vi "Energize.vi"(8 "error in (no error)":errorcluster, 11 "CIFTemplatePlugin in":refnum<class "TemplatePlugin.lvclass">) -> (0 "error out":errorcluster, 3 "CIFTemplatePlugin out":refnum<class "TemplatePlugin.lvclass">)   [LabVIEW 2021, in "TemplatePlugin.lvlib"]
uses:
  TemplatePlugin.lvlib
  Class/TemplatePlugin.lvclass
  D:/dev/CIF-LVCore/src/CIFCore/Class/CIFCorePlugin.lvclass
  CIF-LVCore/src/CIFCore/Class/CIFCorePlugin.lvclass/CIFCorePlugin.ctl
  Class/TemplatePlugin.lvclass/TemplatePlugin.ctl
  <vilib>/CIF Foundation/CIF Utilities/Statistics/I64/Stats_I64_CIF_U.lvclass/Stats_I64_CIF_U.ctl
  CIF-LVCore/src/Channels/CIFChannelMng/CIFChannelMng.lvclass/CIFChannelMng.ctl
  <vilib>/CIF Foundation/CIF Channels Core/CIFChannels/CIFChannels.lvclass/CIFChannels.ctl
  <vilib>/CIF Foundation/CIF Utilities/Time/System Time/Get System Time.vi
  CIF-LVCore/src/CIFCore/Class/SubVIs/Running State Logic.vi
  Class/Dynamic/Execute.vi
  Class/Dynamic/Housekeeping.vi
  CIF-LVCore/src/CIFCore/Class/SubVIs/OOB/Send Core OOB TX.vi
  CIF-LVCore/src/CIFCore/Class/Accessors/Read Energized State.vi
  CIF-LVCore/src/CIFCore/Class/SubVIs/Start Running.vi
  <vilib>/CIF Foundation/CIF Utilities/Time/System Time/LabVIEW Time to TAI Time.vi
  Class/Dynamic/Logic.vi
  CIF-LVCore/src/CIFCore/Class/Accessors/Write Energized State.vi
  CIF-LVCore/src/CIFCore/Class/SubVIs/Sleep.vi
  CIF-LVCore/src/CIFCore/Class/Benchmarking/Benchmark Running.vi
  CIF-LVCore/src/CIFCore/Class/SubVIs/OOB/Read Core OOB RX.vi
  Class/OOB Comm/Read Comm to Main.vi
  Class/OOB Comm/Send Cyclic to gRPC.vi
  CIF-LVCore/src/CIFCore/Class/SubVIs/OOB/Update Status from Benchmarks.vi
  CIF-LVCore/src/Channels/CIFChannelMng/Core/Send Channel List Update.vi
  CIF-LVCore/src/CIFCore/Class/SubVIs/OOB/Send Core OOB TX.vi/074d8088-3ad4-4fdc-9542-b009f1b06b72.vi
  <vilib>/CIF Foundation/CIF Utilities/Time/System Time/Sleep Until Future Time.vi
  CIF-LVCore/src/CIFCore/Class/Channel RW/Read U64.vi
  CIF-LVCore/src/CIFCore/Class/Channel RW/Write U64.vi
  CIF-LVCore/src/CIFCore/Class/Channel RW/Write Double.vi
  CIF-LVCore/src/CIFCore/Class/Channel RW/Read Double.vi
  CIF-LVCore/src/CIFCore/Class/Accessors/Monitor/Write Double 1.vi
  CIF-LVCore/src/CIFCore/Class/Accessors/Monitor/Write U64 1.vi
  CIF-LVCore/src/CIFCore/Class/Accessors/Monitor/Write U64 2.vi
  CIF-LVCore/src/CIFCore/Class/Accessors/Monitor/Write I64 1.vi
  CIF-LVCore/src/CIFCore/Class/Accessors/Monitor/Write I64 2.vi
  CIF-LVCore/src/CIFCore/Class/Accessors/Timestamps/Write Execute TS.vi
  CIF-LVCore/src/CIFCore/Class/Accessors/Timestamps/Write Sleep TS.vi
  <vilib>/Utility/error.llb/Clear Errors.vi
  CIF-LVCore/src/CIFCore/Class/Accessors/Read Sleep Limits (ns).vi
  CIF-LVCore/src/CIFCore/Class/Accessors/Timestamps/Write Target Wake TS.vi
  CIF-LVCore/src/CIFCore/Class/Accessors/Read Plugin Name.vi
  CIF-LVCore/src/CIFCore/Common/Utilities/Add Error.vi
  CIF-LVCore/src/CIFCore/Class/Accessors/Timestamps/Read Running TS.vi
  CIF-LVCore/src/CIFCore/Class/Benchmarking/Reset Delay.vi
  CIF-LVCore/src/CIFCore/Class/Accessors/Read Running Internal Data.vi
  CIF-LVCore/src/CIFCore/Class/Accessors/Read Timing Override.vi
  CIF-LVCore/src/CIFCore/Class/Accessors/Read Common Config.vi
  CIF-LVCore/src/CIFCore/Class/Accessors/Timestamps/Write Housekeeping TS.vi
  <vilib>/CIF Foundation/CIF Utilities/Statistics/I64/X1 minus X0.vi
  <vilib>/CIF Foundation/CIF Utilities/Statistics/I64/Cyclic.vi
  CIF-LVCore/src/CIFCore/Class/Accessors/Timestamps/Read Execute TS.vi
  CIF-LVCore/src/CIFCore/Class/Accessors/Timestamps/Read Housekeeping TS.vi
  CIF-LVCore/src/CIFCore/Class/Accessors/Timestamps/Read Sleep TS.vi
  CIF-LVCore/src/CIFCore/Class/Accessors/Timestamps/Read Target Wake TS.vi
  CIF-LVCore/src/CIFCore/Class/SubVIs/Refresh Stats.vi
  CIF-LVCore/src/CIFCore/Class/SubVIs/OOB/Receive/Read Clock Map.vi
  CIF-LVCore/src/CIFCore/Class/SubVIs/OOB/Receive/Read Connections.vi
  CIF-LVCore/src/Channels/CIFChannelMng/SubVIs/Connect Channel.vi
  CIF-LVCore/src/CIFCore/Class/SubVIs/OOB/Receive/Read Forces.vi
  CIF-LVCore/src/Channels/CIFChannelMng/SubVIs/Force Channel.vi
  CIF-LVCore/src/Channels/CIFChannelMng/SubVIs/Add FIFO Publisher.vi
  CIF-LVCore/src/CIFCore/Class/SubVIs/OOB/Receive/Read Publisher Instance.vi
  CIF-LVCore/src/Channels/CIFChannelMng/Core/Send Publisher Instance Return.vi
  CIF-LVCore/src/Channels/CIFChannelMng/SubVIs/Remove FIFO Publisher.vi
  CIF-LVCore/src/CIFCore/Class/SubVIs/OOB/Read Core OOB RX.vi/a31a91a9-4107-4750-8e0d-44486e9a3a34.vi
  Class/OOB Comm/Read Comm to Main.vi/525c214c-2a6b-4e7b-b3ce-0ad96b412d2f.vi
  Class/OOB Comm/Read Comm to Main.vi/4efb0375-f1de-4191-b03f-44d34e6646cb.vi
  Class/OOB Comm/Send Cyclic to gRPC.vi/0c0f428d-7269-422d-ba27-f9d6fa7232ec.vi
  CIF-LVCore/src/CIFCore/Class/Accessors/Read Refresh.vi
  <vilib>/CIF Foundation/CIF Utilities/Statistics/I64/Get Stats.vi
  CIF-LVCore/src/Channels/CIFChannelMng/Core/Send Channel List Update.vi/463ebf4c-8748-40f9-8ad3-9e61c16a01a6.vi
  <vilib>/CIF Foundation/CIF CIPC/SubVIs/Check Error.vi
  <vilib>/CIF Foundation/CIF CIPC/SubVIs/Notify Of New Write.vi
  <vilib>/CIF Foundation/CIF CIPC/SubVIs/Get dll Path.vi
  <vilib>/CIF Foundation/CIF CIPC/SubVIs/Get Element Write Position.vi
  <vilib>/CIF Foundation/CIF Utilities/Time/SubVIs/Add Error.vi
  <vilib>/CIF Foundation/CIF Utilities/Errors/Append Error Location.vi
  <vilib>/CIF Foundation/CIF Utilities/Statistics/I64/X1 minus X0.vi/dfabcf33-0dbc-4041-80a5-3dc0c86d2989.vi
  <vilib>/CIF Foundation/CIF Utilities/Statistics/I64/Cyclic.vi/dfabcf33-0dbc-4041-80a5-3dc0c86d2989.vi
  CIF-LVCore/src/Channels/CIFChannelMng/Utilities/Get Channel Index by Name.vi
  <vilib>/CIF Foundation/CIF Channels Core/CIFChannels/Accessors/Read Channel State.vi
  <vilib>/CIF Foundation/CIF Channels Core/CIFChannels/Accessors/Read Tag Forced.vi
  CIF-LVCore/src/Channels/CIFChannelMng/SubVIs/Add Error Channel Manager.vi
  CIF-LVCore/src/Channels/CIFChannelMng/Core/Send Publisher Instance Return.vi/9db40550-ae0b-4108-a32d-02e81b824dbe.vi
  CIF-LVCore/src/Channels/CIFChannelMng/SubVIs/Get Original FIFO Channel Name.vi
  <vilib>/CIF Foundation/CIF CIPC/SubVIs/Wait For N Elements Available.vi
  <vilib>/CIF Foundation/CIF CIPC/SubVIs/Get Element Read Position.vi
  <vilib>/CIF Foundation/CIF CIPC/SubVIs/Set Element Read Position.vi
  <vilib>/CIF Foundation/CIF Utilities/Statistics/I64/X1 minus X0.vi/dfabcf33-0dbc-4041-80a5-3dc0c86d2989.vi/9eb60a9a-770f-4d2d-8b3f-8465c267ecc9.vi
  <vilib>/CIF Foundation/CIF Utilities/Statistics/I64/Cyclic.vi/dfabcf33-0dbc-4041-80a5-3dc0c86d2989.vi/9eb60a9a-770f-4d2d-8b3f-8465c267ecc9.vi
  <vilib>/CIF Foundation/CIF Channels Core/ChannelCommon/Utilities/Add Error.vi
  CIF-LVCore/src/CIFCore/Class/Logs/Log Run.vi
  <vilib>/CIF Foundation/CIF CIPC/SubVIs/Get Element Info Variant.vi
  <vilib>/Utility/error.llb/Trim Whitespace.vi
  <vilib>/Utility/error.llb/Error Cluster From Error Code.vi
  <vilib>/CIF Foundation/CIF Channels Core/CIFChannels/Core/Set Force.vi
  <vilib>/CIF Foundation/CIF Channels Core/CIFChannels/CIFChannels.lvclass
  CIF-LVCore/src/CIFCore/Class/CIFCorePlugin.lvclass
  <vilib>/Platform/TimedLoop/XDataNode/XDataNode.xnode
  <vilib>/Platform/TimedLoop/XDataNode/nitl_modes.ctl
  <vilib>/Platform/TimedLoop/XDataNode/XDNodeRunTimeDep.lvlib
  <vilib>/Platform/TimedLoop/XDataNode/wakeup.ctl
  <vilib>/Platform/TimedLoop/XDataNode/timing_clust.ctl
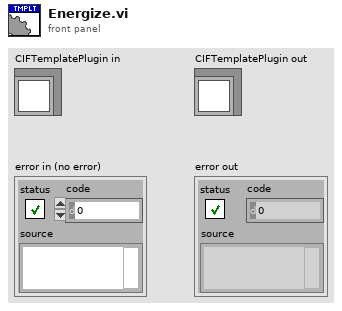
[diagram p1: front panel]
types:
  T1 = typedef "XDNodeRunTimeDep.lvlib/timing_clust.ctl" = cluster{"Expected End [f-1]":u64, "Actual End [f-1]":u64, "Finished Late? [f-1]":bool, "Expected End [i-1]":u64, "Actual End [i-1]":u64, "Finished Late? [i-1]":bool, "Expected Start [i]":u64, "Actual Start [i]":u64, "Expected Start [f]":u64, "Actual Start [f]":u64, "Source Name":string, "Structure Name":string, "Period":i64, "Deadline":i64, "Offset":i64, "Start":i64, "Priority":i32, "Timeout":i32, "Mode":T2, "Wakeup Reason":T3, "Error":errorcluster, "Source Type":string, "Secondary Source Type":string, "Global End Time":u64, "Global Start Time":u64, "Frame Duration":u64, "Iteration Duration":u64, "Assigned CPU":i32, "I/O Scan Engine Mode":u32}
  T2 = typedef "XDNodeRunTimeDep.lvlib/nitl_modes.ctl" = enum32{"No Change", "Process missed periods, maintain original phase", "Discard missed periods, maintain original phase", "Process missed periods, ignore original phase", "Discard missed periods, ignore original phase"}
  T3 = typedef "XDNodeRunTimeDep.lvlib/wakeup.ctl" = enum32{"Normal", "Aborted", "Asynchronous wakeup", "Timing source error", "Timed loop error", "Timeout"}
  T4 = typedef "CIFCorePlugin.lvclass/Prepare State Logic.ctl" = enum16{"Listen", "Prepare", "Error", "Destroy"}
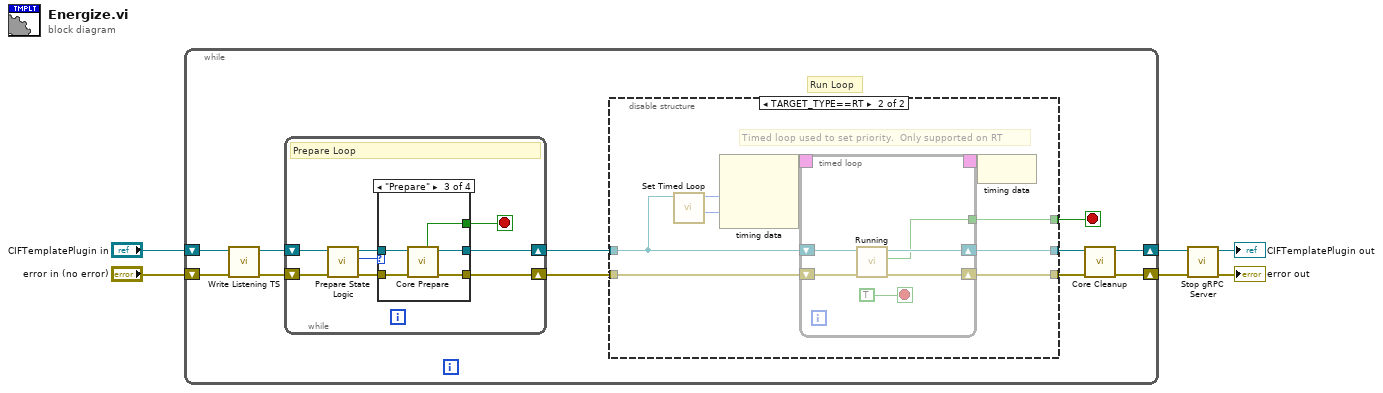
[diagram p0: block diagram]
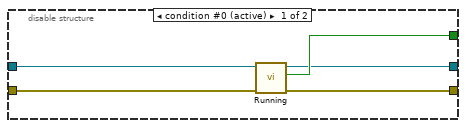
[diagram p2: hidden frame]
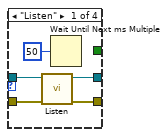
[diagram p3: hidden frame]
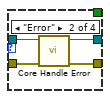
[diagram p4: hidden frame]
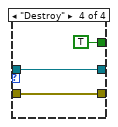
[diagram p5: hidden frame]
diagram:
  n1 = while {
    shift-right: [w17] -> w6
    shift-left: "CIFTemplatePlugin in" -> [w12]
    shift-right: [w16] -> w5
    shift-left: "error in (no error)" -> [w15]
    stop <- w7 stop-if-true
    # "Run Loop"
    n2 = call "Write Listening TS.vi"("error in (no error)"=w15, "CIFCorePlugin in"=w12) -> ("error out"=w13:errorcluster, "CIFCorePlugin out"=w14:refnum<class "TemplatePlugin.lvclass">)  [unwired: 8 in]
    n3 = while {
      shift-right: [w52] -> w11
      shift-left: w14 -> [w45]
      shift-right: [w47] -> w10
      shift-left: w13 -> [w48]
      stop <- w46 stop-if-true
      # "Prepare Loop"
      n4 = call "Prepare State Logic.vi"("error in (no error)"=w48, "CIFCorePlugin in"=w45) -> ("error out"=w49:errorcluster, "Prepare State Logic"=w50:T4, "CIFCorePlugin out"=w51:refnum<class "TemplatePlugin.lvclass">)  [unwired: 7 in]
      n5 = case shown="\"Prepare\"" w50 {
        tunnel: [w53 w61 w66 w69] -> w52
        tunnel: w51 -> [w55 w58 w62 w69]
        tunnel: w49 -> [w56 w59 w63 w68]
        tunnel: [w54 w60 w65 w68] -> w47
        tunnel: [_ _ w64 TRUE ("Transition to Run")] -> w46
        frame "Listen" {
          n6 = call-dynamic "Listen.vi"("error in (no error)"=w56, "CIFTemplatePlugin in"=w55) -> ("error out"=w54:errorcluster, "CIFTemplatePlugin out"=w53:refnum<class "TemplatePlugin.lvclass">)  [unwired: 8 in]
          n7 = Wait Until Next ms Multiple(millisecond multiple=u32 50) -> ()  [unwired: 1 out]
        }
        frame "Error" {
          n8 = call "Core Handle Error.vi"("error in (no error)"=w59, "CIFTemplateNode in"=w58) -> ("error out"=w60:errorcluster, "CIFTemplateNode out"=w61:refnum<class "TemplatePlugin.lvclass">)  [unwired: 8 in]
        }
        frame "Prepare" {
          n9 = call "Core Prepare.vi"("error in (no error)"=w63, "CIFTemplateNode in"=w62) -> ("error out"=w65:errorcluster, "CIFTemplateNode out"=w66:refnum<class "TemplatePlugin.lvclass">, "Transition to Run"=w64:bool)  [unwired: 7 in]
        }
        frame "Destroy" {
        }
      }
    }
    n10 = disable-structure shown="TARGET_TYPE==RT" {
      disable-tunnel: w11 -> [w22 w23]
      disable-tunnel: w10 -> [w21 w29]
      disable-tunnel: [w20 w28] -> w7
      disable-tunnel: [w18 w27] -> w9
      disable-tunnel: [w19 w26] -> w8
      frame condition #0 (active) {
        n11 = call "Running.vi"("error in (no error)"=w21, "CIFTemplatePlugin in"=w22) -> ("error out"=w19:errorcluster, "Destroy"=w20:bool, "CIFTemplatePlugin out"=w18:refnum<class "TemplatePlugin.lvclass">)  [unwired: 7 in]
      }
      frame condition #1 {
        # "Timed loop used to set priority.  Only supported on RT"
        n12 = call "Set Timed Loop.vi"("CIFCorePlugin in"=w23) -> ("Processor"=w24:i32, "Priority"=w25:i32)  [unwired: 9 in]
        n13 = node-c288(w25, w24) -> (w31:T1)  [unwired: 1 in]
        n14 = timed-loop {
          timing: w31 -> [_]
          timing-out: [_] -> w30
          shift-right: [w33] -> w27
          shift-left: w23 -> [w36]
          shift-right: [w34] -> w26
          shift-left: w29 -> [w35]
          tunnel: [w32] -> w28
          stop <- TRUE stop-if-true
          n15 = call "Running.vi"("error in (no error)"=w35, "CIFTemplatePlugin in"=w36) -> ("error out"=w34:errorcluster, "Destroy"=w32:bool, "CIFTemplatePlugin out"=w33:refnum<class "TemplatePlugin.lvclass">)  [unwired: 7 in]
        }
        n16 = node-c288(w30) -> ()
      }
    }
    n17 = call "Core Cleanup.vi"("error in (no error)"=w8, "CIFTemplateNode in"=w9) -> ("error out"=w16:errorcluster, "CIFTemplateNode out"=w17:refnum<class "TemplatePlugin.lvclass">)  [unwired: 8 in]
  }
  n18 = call "Stop gRPC Server.vi"("error in (no error)"=w5, "CIFCorePlugin in"=w6) -> ("error out"=→"error out":errorcluster, "CIFCorePlugin out"=→"CIFTemplatePlugin out":refnum<class "TemplatePlugin.lvclass">)  [unwired: 8 in]
